vi "get recursive datatype.vi"(8 "error in":errorcluster, 10 "Type Descriptor":T1) -> (0 "error out":errorcluster, 2 "Recursive Datatype":T2[](array[typedef]))   [LabVIEW 2009]
doc: "Returns an array representing the datatype stored within the variant. Can be used to determine if one variant is the same datatype as another (or can easily be converted). This vi calls itself recursively."
uses:
  datatype.ctl
  <userlib>/_OpenG.lib/lvdata/lvdata.llb/Type Descriptor__ogtk.ctl
panel:
  in  "for recursive call to self":refnum<vi>
  # "Get Default Data from TD.vi\n\nReturns default data of the type defined by the TD.  This vi calls itself recurs\n\nPlease visit http://www.OpenG.org to learn about the\nOpen Source LabVIEW software movement.\n\nNOTICE -- YOU MUST LEAVE THIS NOTICE IN PLACE.  PER THE TERMS OF THE LICENSE BELOW, YOU MAY SUBLICENSE THIS SOFTWARE \nIN ANY WAY THAT DOES NOT CONFLICT WITH THIS LICENSE.\n\n### BSD License (http://www.opensource.org/licenses/bsd-license.php) Begin ###\n \nCopyright (c) 2002, Jean-Pierre Drolet <drolet_jp@hotmail.com>\nCopyright (c) 2002-2006, Jim Kring <jim@jimkring.com>\n\nAll rights reserved.\n\nRedistribution and use in source and binary forms, with or without modification, are permitted provided that the following conditions are met:\n\n    * Redistributions of source code must retain the above copyright notice, this list of conditions and the following disclaimer.\n    * Redistributions in binary form must reproduce the above copyright notice, this list of conditions and the following disclaimer in the \n       documentation and/or other materials provided with the distribution.\n    * Neither the name of SciWare, James Kring, Inc., nor the names of its contributors may be used to endorse or promote products derived \n       from this software without specific prior written permission.\n\nTHIS SOFTWARE IS PROVIDED BY THE COPYRIGHT HOLDERS AND CONTRIBUTORS \"AS IS\" AND ANY EXPRESS OR IMPLIED WARRANTIES, \nINCLUDING, BUT NOT LIMITED TO, THE IMPLIED WARRANTIES OF MERCHANTABILITY AND FITNESS FOR A PARTICULAR PURPOSE ARE \nDISCLAIMED. IN NO EVENT SHALL THE COPYRIGHT OWNER OR CONTRIBUTORS BE LIABLE FOR ANY DIRECT, INDIRECT, INCIDENTAL,\n SPECIAL, EXEMPLARY, OR CONSEQUENTIAL DAMAGES (INCLUDING, BUT NOT LIMITED TO, PROCUREMENT OF SUBSTITUTE GOODS OR \nSERVICES; LOSS OF USE, DATA, OR PROFITS; OR BUSINESS INTERRUPTION) HOWEVER CAUSED AND ON ANY THEORY OF LIABILITY, \nWHETHER IN CONTRACT, STRICT LIABILITY, OR TORT (INCLUDING NEGLIGENCE OR OTHERWISE) ARISING IN ANY WAY OUT OF THE USE \nOF THIS SOFTWARE, EVEN IF ADVISED OF THE POSSIBILITY OF SUCH DAMAGE.\n\n### BSD License End ###"
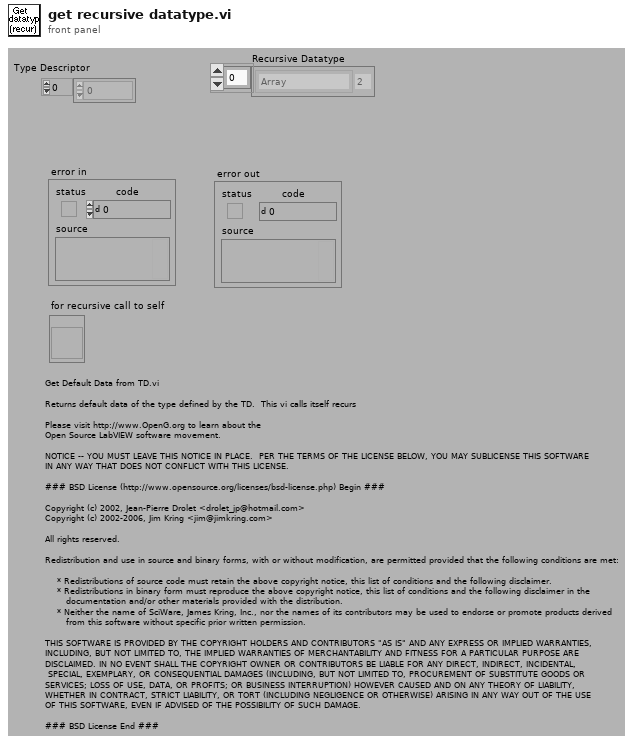
[diagram p1: front panel]
types:
  T1 = typedef "Type Descriptor__ogtk.ctl" = i16[]
  T2 = typedef "datatype.ctl" = enum8{"<Null>", "Cluster", "Array", "Boolean", "Path", "String", "Number", "Refnum", "Waveform", "Pict", "DAQ"}
  T3 = typedef "Type Descriptor Header__ogtk.ctl" = cluster{"length":u16, "private":u8, "type":T4, "# elements":u16}
  T4 = typedef "Type Descriptor Enumeration__ogtk.ctl" = enum8{"<Null>", "I8", "I16", "I32", "I64", "U8", "U16", "U32", "U64", "SGL", "DBL", "EXT", "CSG", "CDB", "CXT", "0x0F", "0x10", "0x11", "0x12", "0x13", "0x14", "Enum U8", "Enum U16", "Enum U32", "Enum U64", "SGL PQ", "DBL PQ", "EXT PQ", "CSG PQ", "CDB PQ", "CXT PQ", "0x1F", "0x20", "Boolean", "0x22", "0x23", "0x24", "0x25", "0x26", "0x27", "0x28", "0x29", "0x2A", "0x2B", "0x2C", "0x2D", "0x2E", "0x2F", "String", "0x31", "Path", "Pict", "0x34", "0x35", "0x36", "DAQ", "0x38", "0x39", "0x3A", "0x3B", "0x3C", "0x3D", "0x3E", "0x3F", "Array", "0x41", "0x42", "0x43", "0x44", "0x45", "0x46", "0x47", "0x48", "0x49", "0x4A", "0x4B", "0x4C", "0x4D", "0x4E", "0x4F", "Cluster", "0x51", "0x52", "Variant", "Waveform", "0x55", "0x56", "0x57", "0x58", "0x59", "0x5A", "0x5B", "0x5C", "0x5D", "0x5E", "0x5F", "0x60", "0x61", "0x62", "0x63", "0x64", "0x65", "0x66", "0x67", "0x68", "0x69", "0x6A", "0x6B", "0x6C", "0x6D", "0x6E", "0x6F", "Refnum"}
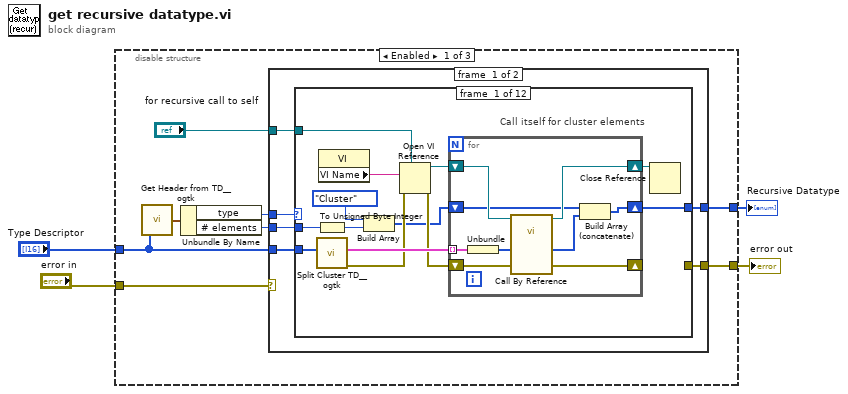
[diagram p0: block diagram]
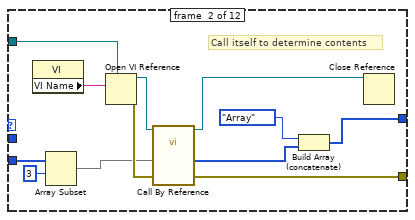
[diagram p2: hidden frame]
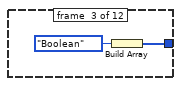
[diagram p3: hidden frame]
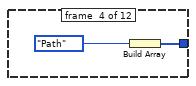
[diagram p4: hidden frame]
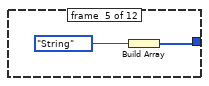
[diagram p5: hidden frame]
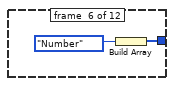
[diagram p6: hidden frame]
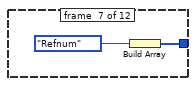
[diagram p7: hidden frame]
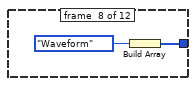
[diagram p8: hidden frame]
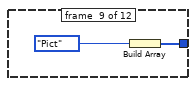
[diagram p9: hidden frame]
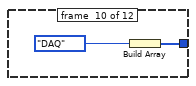
[diagram p10: hidden frame]
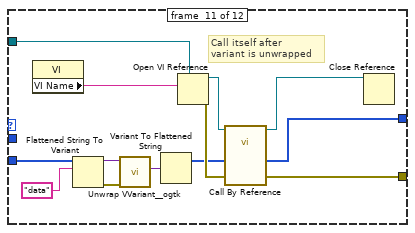
[diagram p11: hidden frame]
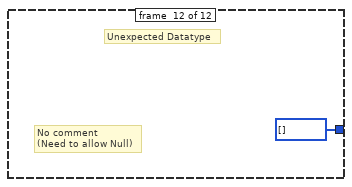
[diagram p12: hidden frame]
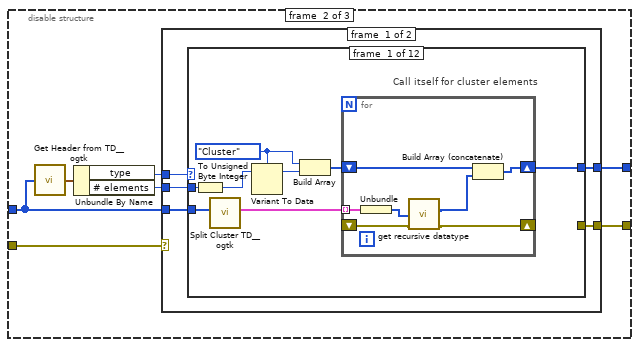
[diagram p14: hidden frame]
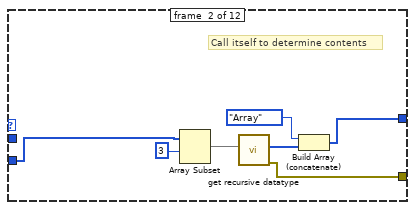
[diagram p15: hidden frame]
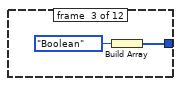
[diagram p16: hidden frame]
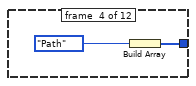
[diagram p17: hidden frame]
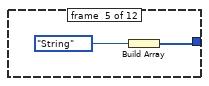
[diagram p18: hidden frame]
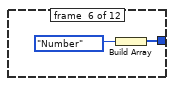
[diagram p19: hidden frame]
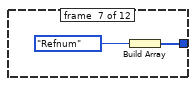
[diagram p20: hidden frame]
diagram:
  n1 = disable-structure shown="Enabled" {
    disable-tunnel: "error in" -> [w12 w90 _]
    disable-tunnel: "Type Descriptor" -> [w11 w89 _]
    disable-tunnel: [w10 w88 _] -> w2
    disable-tunnel: [w6 w84 _] -> w1
    frame #0 {
      n2 = call <userlib>:"Get Header from TD__ogtk.vi"("Type Descriptor"=w11) -> ("Type Descriptor Header"=w9:T3)
      n3 = Unbundle By Name(w9) -> ("type"=w8:T4, "# elements"=w7:u16)
      n4 = case shown="No Error" w12 {
        selector: w12 -> [_ w83]
        tunnel: w8 -> [w18 _]
        tunnel: [w17 w83] -> w10
        tunnel: w11 -> [w16 _]
        tunnel: w7 -> [w15 _]
        tunnel: [w14 _] -> w6
        tunnel: "for recursive call to self" -> [w13 _]
        frame #0 {
          n5 = case shown="\"Array\"" w18 {
            tunnel: [_ w47 _ _ _ _ _ _ _ _ w75 _] -> w17
            tunnel: w16 -> [w26 w45 _ _ _ _ _ _ _ _ w72 _]
            tunnel: w15 -> [w23 _ _ _ _ _ _ _ _ _ _ _]
            tunnel: [w25 w41 w53 w55 w57 w59 w61 w63 w65 w67 w76 u8[] [] ("Datatype")] -> w14
            tunnel: w13 -> [w20 w48 _ _ _ _ _ _ _ _ w77 _]
            frame #0 {
              # "Call itself for cluster elements"
              n6 = To Unsigned Byte Integer(number=w23) -> (unsigned 8bit integer=w22:u8)
              n7 = call "Split Cluster TD__ogtk.vi"("Type Descriptor"=w26) -> ("error out"=w24:errorcluster, "Type Descriptors"=w31:cluster{"Type Descriptor":T1}[])  [unwired: 1 in, 8 out]
              n8 = property class="VI"() -> ("VI Name"=w30:string)  [unwired: 2 in, 2 out]
              n9 = Build Array(datatype."Cluster" ("Datatype"), w22) -> (w21:u8[])
              n10 = Open VI Reference(type specifier VI Refnum (for type only)=w20, vi path=w30, error in (no error)=w24) -> (vi reference=w29:refnum<vi>, error out=w27:errorcluster)  [unwired: 1 in, 2 out]
              n11 = for {
                tunnel: w31 -> [w40] mode=indexing
                shift-right: [w37] -> _
                shift-left: w27 -> [w38]
                shift-right: [w35] -> w28
                shift-left: w29 -> [w36]
                shift-right: [w33] -> w25
                shift-left: w21 -> [w32]
                n12 = Unbundle(w40) -> ("Type Descriptor"=w39:T1)
                n13 = call-by-ref "?"(reference=w36, "error in"=w38, "Type Descriptor"=w39) -> (reference out=w35:refnum<vi>, "error out"=w37:errorcluster, "Datatype"=w34:u8[])  [unwired: 9 in, 1 out]
                n14 = Build Array (concatenate)(w32, w34) -> (w33:u8[])
              }
              n15 = Close Reference(reference=w28) -> ()  [unwired: 1 in, 1 out]
            }
            frame #1 {
              # "Call itself to determine contents"
              n16 = property class="VI"() -> ("VI Name"=w52:string)  [unwired: 2 in, 2 out]
              n17 = Array Subset(array=w45, index=3) -> (w44:T1)  [unwired: 1 in]
              n18 = Open VI Reference(type specifier VI Refnum (for type only)=w48, vi path=w52) -> (vi reference=w51:refnum<vi>, error out=w49:errorcluster)  [unwired: 2 in, 2 out]
              n19 = call-by-ref "?"(reference=w51, "error in"=w49, "Type Descriptor"=w44) -> (reference out=w50:refnum<vi>, "error out"=w47:errorcluster, "Datatype"=w43:u8[])  [unwired: 9 in, 1 out]
              n20 = Build Array (concatenate)(datatype."Array" ("Datatype"), w43) -> (w41:u8[])
              n21 = Close Reference(reference=w50) -> ()  [unwired: 1 in, 1 out]
            }
            frame #2 {
              n22 = Build Array(datatype."Boolean" ("Datatype")) -> (w53:T2[])
            }
            frame #3 {
              n23 = Build Array(datatype."Path" ("Datatype")) -> (w55:T2[])
            }
            frame #4 {
              n24 = Build Array(datatype."String" ("Datatype")) -> (w57:T2[])
            }
            frame #5 {
              n25 = Build Array(datatype."Number" ("Datatype")) -> (w59:T2[])
            }
            frame #6 {
              n26 = Build Array(datatype."Refnum" ("Datatype")) -> (w61:T2[])
            }
            frame #7 {
              n27 = Build Array(datatype."Waveform" ("Datatype")) -> (w63:T2[])
            }
            frame #8 {
              n28 = Build Array(datatype."Pict" ("Datatype")) -> (w65:T2[])
            }
            frame #9 {
              n29 = Build Array(datatype."DAQ" ("Datatype")) -> (w67:T2[])
            }
            frame #10 {
              # "Call itself after\nvariant is unwrapped"
              n30 = property class="VI"() -> ("VI Name"=w81:string)  [unwired: 2 in, 2 out]
              n31 = Flattened String To Variant(6:"data", 7:w72) -> (0:w74:errorcluster, 3:w73:variant)  [unwired: 1 in]
              n32 = call "Unwrap VVariant__ogtk.vi"("error in (no error)"=w74, "VVariant"=w73) -> ("Variant"=w71:variant)  [unwired: 9 out]
              n33 = Variant To Flattened String(Variant=w71) -> (1:w70:i16[])  [unwired: 1 out]
              n34 = Open VI Reference(type specifier VI Refnum (for type only)=w77, vi path=w81) -> (vi reference=w80:refnum<vi>, error out=w78:errorcluster)  [unwired: 2 in, 2 out]
              n35 = call-by-ref "?"(reference=w80, "error in"=w78, "Type Descriptor"=w70) -> (reference out=w79:refnum<vi>, "error out"=w75:errorcluster, "Datatype"=w76:u8[])  [unwired: 9 in, 1 out]
              n36 = Close Reference(reference=w79) -> ()  [unwired: 1 in, 1 out]
            }
            frame #11 {
              # "No comment\n(Need to allow Null)"
              # "Unexpected Datatype"
            }
          }
        }
        frame #1 {
          (unwired) variant
        }
      }
    }
    frame #1 {
      n37 = call <userlib>:"Get Header from TD__ogtk.vi"("Type Descriptor"=w89) -> ("Type Descriptor Header"=w87:T3)
      n38 = Unbundle By Name(w87) -> ("type"=w86:T4, "# elements"=w85:u16)
      n39 = case shown="No Error" w90 {
        selector: w90 -> [_ w143]
        tunnel: w86 -> [w95 _]
        tunnel: [w94 w143] -> w88
        tunnel: w89 -> [w93 _]
        tunnel: w85 -> [w92 _]
        tunnel: [w91 _] -> w84
        frame #0 {
          n40 = case shown="\"Cluster\"" w95 {
            tunnel: [_ w112 _ _ _ _ _ _ _ _ w134 _] -> w94
            tunnel: w93 -> [w102 w116 _ _ _ _ _ _ _ _ w139 _]
            tunnel: w92 -> [w100 _ _ _ _ _ _ _ _ _ _ _]
            tunnel: [w101 w114 w118 w120 w122 w124 w126 w128 w130 w132 w135 w142] -> w91
            frame #0 {
              w97 = datatype."Cluster" ("Datatype")
              # "Call itself for cluster elements"
              n41 = To Unsigned Byte Integer(number=w100) -> (unsigned 8bit integer=w98:u8)
              n42 = call "Split Cluster TD__ogtk.vi"("Type Descriptor"=w102) -> ("Type Descriptors"=w103:cluster{"Type Descriptor":T1}[])  [unwired: 1 in, 9 out]
              n43 = Variant To Data(Variant=w98, type=w97) -> (data=w96:T2)  [unwired: 1 in, 1 out]
              n44 = Build Array(w97, w96) -> (w99:T2[])
              n45 = for {
                tunnel: w103 -> [w110] mode=indexing
                shift-right: [w104] -> _
                shift-left: _ -> [w105]
                shift-right: [w109] -> w101
                shift-left: w99 -> [w108]
                n46 = Unbundle(w110) -> ("Type Descriptor"=w107:T1)
                n47 = call "get recursive datatype.vi"("error in"=w105, "Type Descriptor"=w107) -> ("error out"=w104:errorcluster, "Recursive Datatype"=w106:T2[])  [unwired: 8 in]
                n48 = Build Array (concatenate)(w108, w106) -> (w109:T2[])
              }
            }
            frame #1 {
              # "Call itself to determine contents"
              n49 = Array Subset(array=w116, index=3) -> (w113:T1)  [unwired: 1 in]
              n50 = call "get recursive datatype.vi"("Type Descriptor"=w113) -> ("error out"=w112:errorcluster, "Recursive Datatype"=w111:T2[])  [unwired: 9 in]
              n51 = Build Array (concatenate)(datatype."Array" ("Datatype"), w111) -> (w114:T2[])
            }
            frame #2 {
              n52 = Build Array(datatype."Boolean" ("Datatype")) -> (w118:T2[])
            }
            frame #3 {
              n53 = Build Array(datatype."Path" ("Datatype")) -> (w120:T2[])
            }
            frame #4 {
              n54 = Build Array(datatype."String" ("Datatype")) -> (w122:T2[])
            }
            frame #5 {
              n55 = Build Array(datatype."Number" ("Datatype")) -> (w124:T2[])
            }
            frame #6 {
              n56 = Build Array(datatype."Refnum" ("Datatype")) -> (w126:T2[])
            }
            frame #7 {
              n57 = Build Array(datatype."Waveform" ("Datatype")) -> (w128:T2[])
            }
            frame #8 {
              n58 = Build Array(datatype."Pict" ("Datatype")) -> (w130:T2[])
            }
            frame #9 {
              n59 = Build Array(datatype."DAQ" ("Datatype")) -> (w132:T2[])
            }
            frame #10 {
              # "Call itself after\nvariant is unwrapped"
              n60 = Flattened String To Variant(6:"data", 7:w139) -> (0:w141:errorcluster, 3:w140:variant)  [unwired: 1 in]
              n61 = call "Unwrap VVariant__ogtk.vi"("error in (no error)"=w141, "VVariant"=w140) -> ("Variant"=w138:variant)  [unwired: 9 out]
              n62 = Variant To Flattened String(Variant=w138) -> (1:w136:i16[])  [unwired: 1 out]
              n63 = call "get recursive datatype.vi"("Type Descriptor"=w136) -> ("error out"=w134:errorcluster, "Recursive Datatype"=w135:T2[])  [unwired: 9 in]
            }
            frame #11 {
              w142 = T2[] [] items=["<Null>", "Cluster", "Array", "Boolean", "Path", "String", "Number", "Refnum", "Waveform", "Pict", "DAQ"] ("Datatype")
              # "No comment\n(Need to allow Null)"
              # "Unexpected Datatype"
            }
          }
        }
        frame #1 {
          (unwired) variant
        }
      }
    }
    frame #2 {
    }
  }
  "error out" <- w2
  "Recursive Datatype" <- w1
